vi "CreateButtonBarFlow.vi"(6 "ShowLegend":bool=TRUE, 9 "Simplified":bool, 10 "TargetFolder":path, 11 "Path":path) -> (2 "Uniques":T1, 3 "PlantUMLText":string)   [LabVIEW 2021, in "ButtonBarFlow.lvlib"]
uses:
  ButtonBarFlow.lvlib
  TAFAOModule_GUI_VerticalButtonBar/VerticalButtonBar/ButtonCollection/ButtonCollection.lvclass
panel:
  in  "Orientation":enum16{"Horizonal", "Vertical"}(ring)
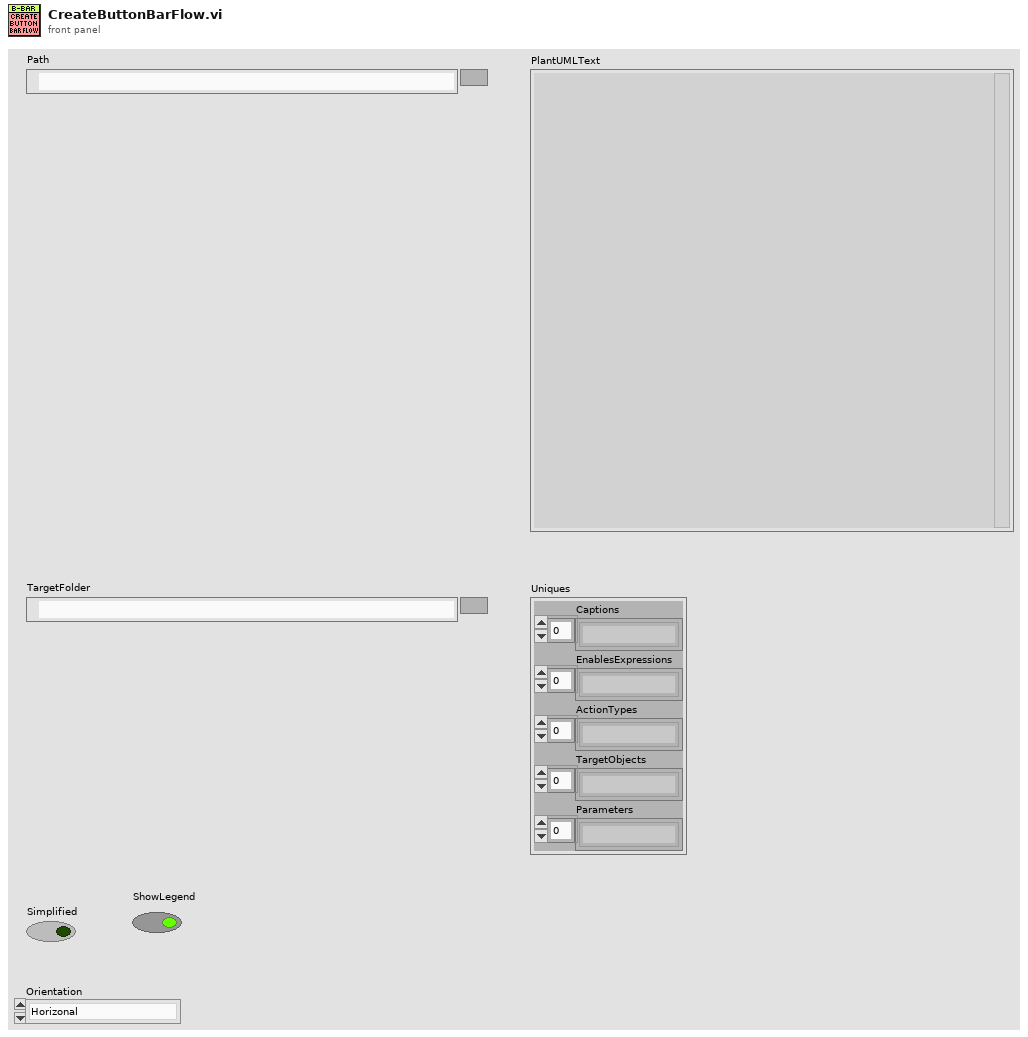
[diagram p1: front panel]
types:
  T1 = cluster{"Captions":string[], "EnablesExpressions":string[], "ActionTypes":string[], "TargetObjects":string[], "Parameters":string[]}
  T2 = typedef "ButtonCollection.lvclass/ButtonDefinition.ctl" = cluster{"ThisNavigationName":string, "ButtonLabel":string, "Caption":string, "Tooltip":string, "EnabledExpression":string, "Actions":cluster{"ActionType":string, "TargetObject":string, "Parameter":string, "WaitUntilDone":bool}[], "NextNavigationName":string}
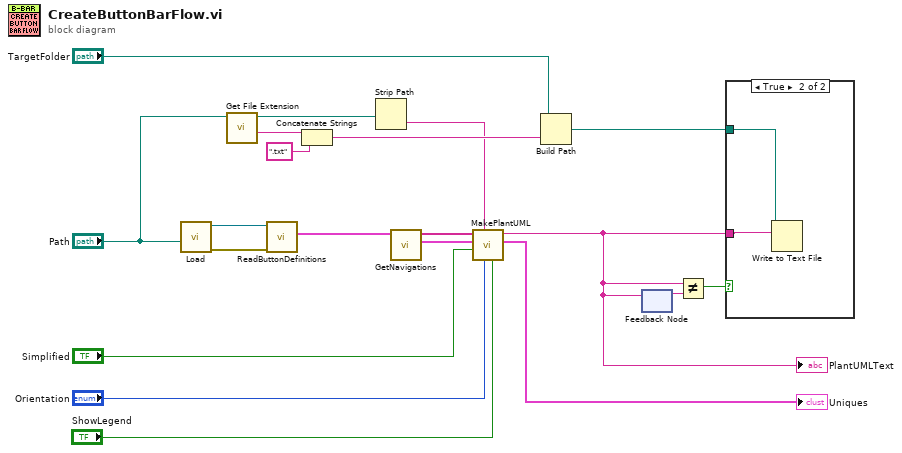
[diagram p0: block diagram]
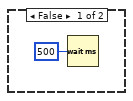
[diagram p2: hidden frame]
diagram:
  n1 = call "Load.vi"("Path"="Path") -> ("ErrorOut"=w19:errorcluster, "ObjectOut"=w18:refnum<class "ButtonCollection.lvclass">)  [unwired: 9 in]
  n2 = call <vilib>:"Get File Extension.vi"("file"="Path") -> ("filename without extension"=w16:string)  [unwired: 6 in, 4 out]
  n3 = call-dynamic "ReadButtonDefinitions.vi"("ErrorIn"=w19, "ObjectIn"=w18) -> ("ButtonDefinitions"=w17:T2[])  [unwired: 7 in, 2 out]
  n4 = Concatenate Strings(w16, ".txt" ("string")) -> (w14:string)
  n5 = Strip Path(path="Path") -> (name=w7:string)  [unwired: 1 out]
  n6 = call "GetNavigations.vi"("ButtonDefinitions"=w17) -> ("Array"=w10:cluster{T2[]}[], "Navigations"=w9:string[])  [unwired: 9 in]
  n7 = call "MakePlantUML.vi"("ShowLegend"="ShowLegend", "Orientation"="Orientation", "DiagramName"=w7, "Simplified"="Simplified", "NavigationsDetails"=w10, "NavigationNames"=w9) -> ("Uniques"=→"Uniques":T1, "PlantUMLText"=w5:string)  [unwired: 4 in]
  "PlantUMLText" <- w5
  n8 = Build Path(base path="TargetFolder", name or relative path=w14) -> (appended path=w13:path)
  n9 = feedback-in #1(w5) -> ()
  n10 = feedback #1() -> (w12:string)  [unwired: 1 in]
  n11 = Not Equal?(x=w5, y=w12) -> (x != y?=w11:bool)
  n12 = case shown="True" w11 {
    tunnel: w13 -> [_ w22]
    tunnel: w5 -> [_ w21]
    frame False {
      n13 = Wait (ms)(milliseconds to wait=u32 500) -> ()  [unwired: 1 out]
    }
    frame True {
      n14 = Write to Text File(file (use dialog)=w22, text=w21) -> ()  [unwired: 2 in, 3 out]
    }
  }
